vi "Read JSONMessage.vi"(8 "error in (no error)":errorcluster, 11 "IJsonMessageHandler in":refnum<class "IJsonMessageHandler.lvclass">) -> (0 "error out":errorcluster, 2 "wamplv.lvlib:JSONMessage.lvclass":refnum<class "JSONMessage.lvclass">, 3 "IJsonMessageHandler out":refnum<class "IJsonMessageHandler.lvclass">)   [LabVIEW 2020, in "wamplv.lvlib" / "IJsonMessageHandler.lvclass"]
uses:
  IJsonMessageHandler.lvclass
  IJsonMessageHandler.lvclass/IJsonMessageHandler.ctl
  SerialisedMessages/JSONMessage/JSONMessage.lvclass
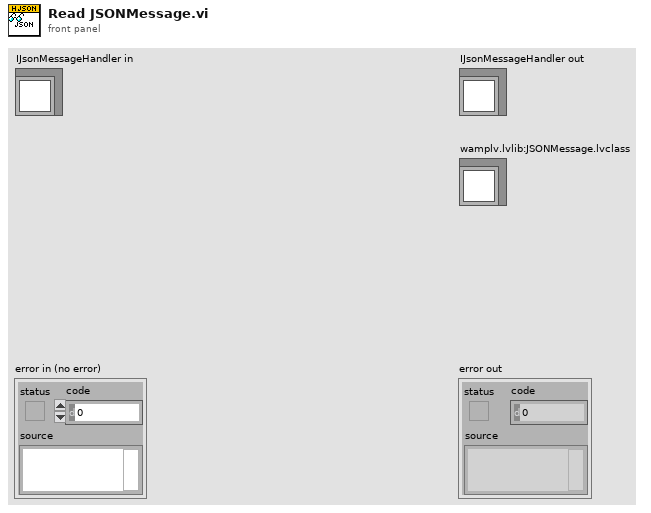
[diagram p1: front panel]
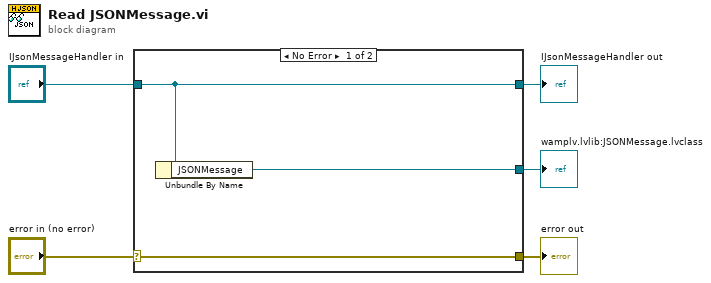
[diagram p0: block diagram]
diagram:
  n1 = case shown="No Error" "error in (no error)" {
    selector: "error in (no error)" -> [w8 w9]
    tunnel: [w8 w9] -> w4
    tunnel: [w7 w10] -> w2
    tunnel: "IJsonMessageHandler in" -> [w7 w10]
    tunnel: [w6 _] -> w1
    frame No Error {
      n2 = Unbundle By Name(w7) -> ("JSONMessage"=w6:refnum<class "JSONMessage.lvclass">)
    }
    frame Error {
    }
  }
  "error out" <- w4
  "IJsonMessageHandler out" <- w2
  "wamplv.lvlib:JSONMessage.lvclass" <- w1
